vi "Untitled 276.vi"() -> ()   [LabVIEW 2026]
uses:
  <vilib>/rvi/interface/nirviOpenFPGA/nirviOpenFPGA.xnode
  <vilib>/rvi/interface/nirviReadWriteControl/nirviReadWriteControl.xnode
  <vilib>/rvi/interface/nirviMethod/nirviMethod.xnode
  <vilib>/FPGAPlugInAG/Dynamic/niLvFpga_Abort_Dynamic.vi
  FPGA Bitfiles/normbuttonpress_FPGATarget_ButtonPitchTest_p7b-oCOOzzg.lvbitx
  Downloads/Button Pitch Test.vi
  <vilib>/FPGAPlugInAG/cRIO-9047/niLvFpga_Open_cRIO-9047.vi
  <vilib>/rvi/interface/common/dynamic/niFpgaDynamicAddResources.vi
  NiFpgaLv.dll
  <vilib>/Utility/error.llb/Error Cluster From Error Code.vi
  <vilib>/rvi/interface/Simulation/niFpgaSimulationCallBeginRW.vi
  <vilib>/rvi/errors/niLvFpgaAdjustHostInterfaceError.vi
panel:
  in  "stop":bool
  in  "duty\ncycle%":dbl
  in  "f":dbl
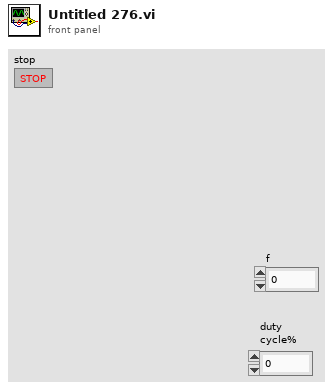
[diagram p1: front panel]
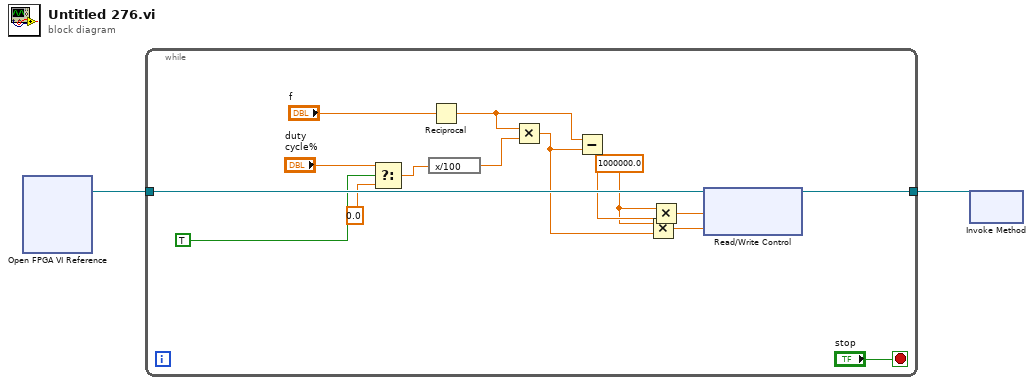
[diagram p0: block diagram]
diagram:
  n1 = xnode "Open FPGA VI Reference"() -> ("FPGA VI Reference Out"=w2:refnum<k20>)  [unwired: 2 in, 1 out]
  n2 = while {
    tunnel: w2 -> [w17]
    tunnel: [w6] -> w1
    stop <- "stop" stop-if-true
    w8 = 1000000.0 ("x")
    n3 = Select(t="duty\ncycle%", s=TRUE ("Boolean"), f=0.0) -> (s? t:f=w5:dbl)
    n4 = expression code="x/100"(w5) -> (w14:dbl)
    n5 = Reciprocal(x="f") -> (1/x=w13:dbl)
    n6 = Multiply(x=w13, y=w14) -> (x*y=w12:dbl)
    n7 = Subtract(x=w13, y=w12) -> (x-y=w11:dbl)
    n8 = Multiply(x=w8, y=w12) -> (x*y=w9:dbl)
    n9 = Multiply(x=w8, y=w11) -> (x*y=w10:dbl)
    n10 = xnode "Read/Write Control"("FPGA VI Reference In"=w17, "Duty Cycle Off"=w10, "Duty Cycle On"=w9) -> ("FPGA VI Reference Out"=w6:refnum<k20>)  [unwired: 1 in, 1 out]
  }
  n11 = xnode "Invoke Method"("FPGA VI Reference In"=w1) -> ()  [unwired: 1 in, 2 out]
